vi "EnvCoverRT.vi"(7 "Out limit":bool, 8 "error in (no error)":errorcluster, 9 "ms timeout (0)":i32, 10 "Status in":enum16{"In", "Moving", "Out", "Wait"}(ring), 11 "In limit":bool) -> (0 "error out":errorcluster, 2 "Ready?":bool, 3 "Status out":enum16{"In", "Moving", "Out", "Wait"}(ring))   [LabVIEW 2015]
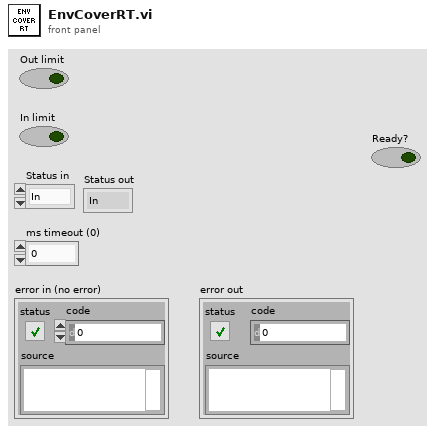
[diagram p1: front panel]
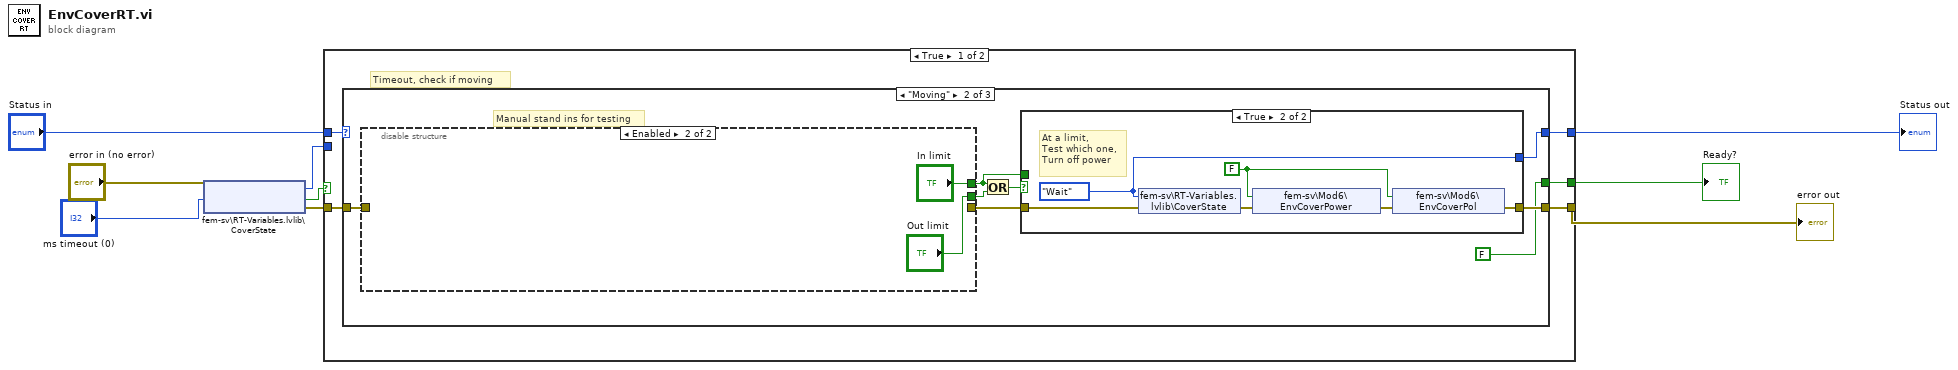
[diagram p0: block diagram]
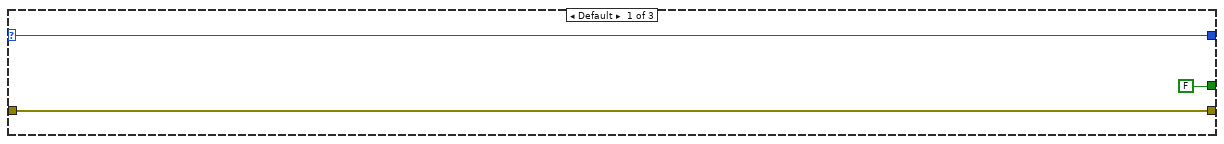
[diagram p2: hidden frame]
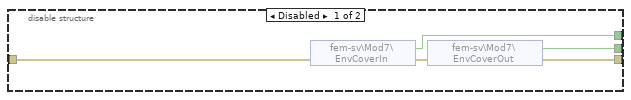
[diagram p3: hidden frame]
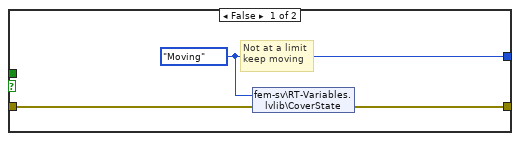
[diagram p4: hidden frame]
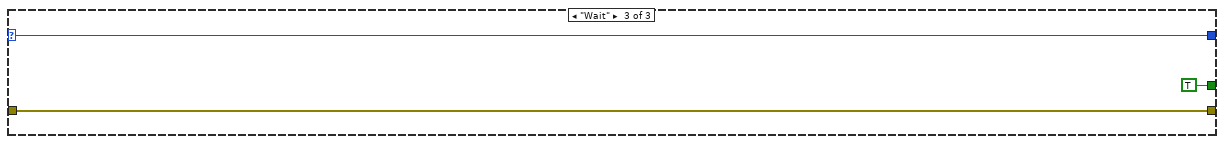
[diagram p5: hidden frame]
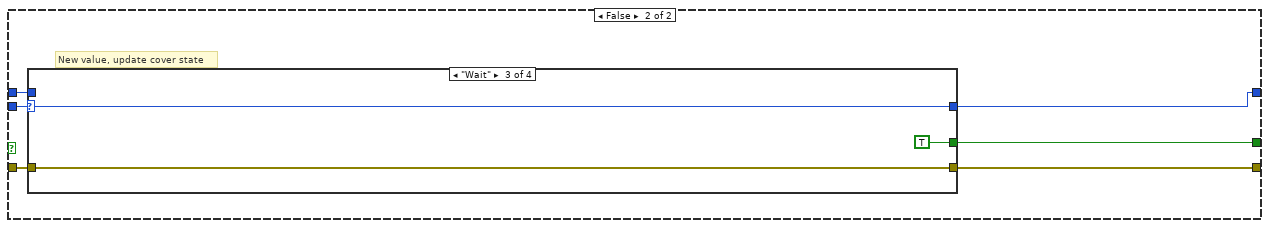
[diagram p6: hidden frame]
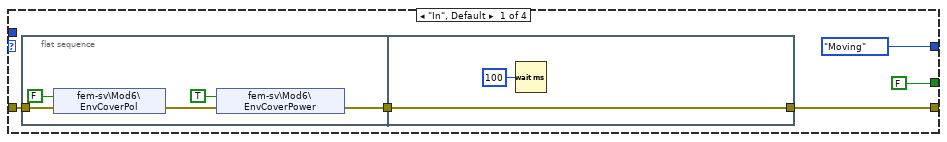
[diagram p7: hidden frame]
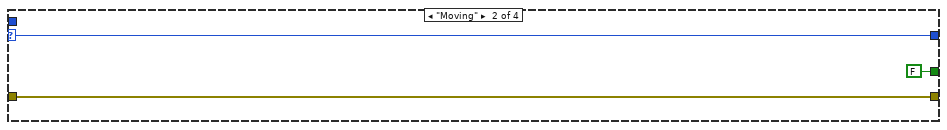
[diagram p8: hidden frame]
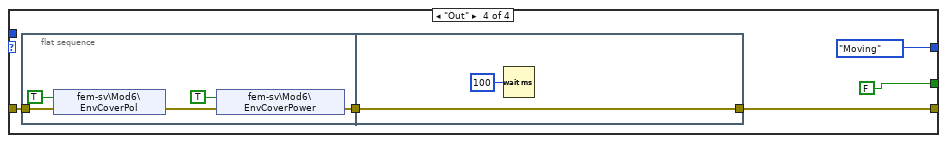
[diagram p9: hidden frame]
diagram:
  n1 = shared-variable "fem-sv\\RT-Variables.lvlib\\CoverState"(error in="error in (no error)", "ms timeout (0)") -> (w5:enum16{"In", "Moving", "Out", "Wait"}, error out=w6:errorcluster, w4:bool)
  n2 = case shown="True" w4 {
    tunnel: [w14 w50] -> w8
    tunnel: "Status in" -> [w11 w49]
    tunnel: w5 -> [_ w48]
    tunnel: w6 -> [w13 w46]
    tunnel: [w12 w47] -> w7
    tunnel: [w10 w45] -> w1
    frame True {
      # "Timeout, check if moving"
      n3 = case shown="\"Moving\"" w11 {
        selector: w11 -> [w17 _ w43]
        tunnel: [w17 w19 w43] -> w14
        tunnel: w13 -> [w16 w23 w42]
        tunnel: [w16 w20 w42] -> w12
        tunnel: [FALSE FALSE TRUE] -> w10
        frame Default {
        }
        frame "Moving" {
          # "Manual stand ins for testing"
          n4 = disable-structure shown="Enabled" {
            disable-tunnel: [w30 "In limit"] -> w24
            disable-tunnel: w23 -> [w29 _]
            disable-tunnel: [w28 "Out limit"] -> w22
            disable-tunnel: [w26 _] -> w21
            frame Disabled {
              n5 = shared-variable "fem-sv\\Mod7\\EnvCoverIn"(error in=w29) -> (w30:bool, error out=w27:errorcluster)
              n6 = shared-variable "fem-sv\\Mod7\\EnvCoverOut"(error in=w27) -> (w28:bool, error out=w26:errorcluster)
            }
            frame Enabled {
            }
          }
          n7 = Or(x=w24, y=w22) -> (x .or. y?=w25:bool)
          n8 = case shown="True" w25 {
            tunnel: w24 -> [_ _]
            tunnel: w21 -> [w35 w41]
            tunnel: [w34 w39] -> w20
            tunnel: [w33 w36] -> w19
            frame False {
              w33 = enum16{"In", "Moving", "Out", "Wait"}."Moving" ("CoverState")
              # "Not at a limit\nkeep moving"
              n9 = shared-variable "fem-sv\\RT-Variables.lvlib\\CoverState"(w33, error in=w35) -> (error out=w34:errorcluster)
            }
            frame True {
              w36 = enum16{"In", "Moving", "Out", "Wait"}."Wait" ("CoverState")
              w37 = FALSE ("EnvCoverPower")
              # "At a limit,\nTest which one,\nTurn off power"
              n10 = shared-variable "fem-sv\\RT-Variables.lvlib\\CoverState"(w36, error in=w41) -> (error out=w38:errorcluster)
              n11 = shared-variable "fem-sv\\Mod6\\EnvCoverPower"(w37, error in=w38) -> (error out=w40:errorcluster)
              n12 = shared-variable "fem-sv\\Mod6\\EnvCoverPol"(w37, error in=w40) -> (error out=w39:errorcluster)
            }
          }
        }
        frame "Wait" {
        }
      }
    }
    frame False {
      # "New value, update cover state"
      n13 = case shown="\"Wait\"" w48 {
        selector: w48 -> [_ w64 w68 _]
        tunnel: [enum16{"In", "Moving", "Out", "Wait"}."Moving" ("Status") w64 w68 enum16{"In", "Moving", "Out", "Wait"}."Moving" ("Status")] -> w50
        tunnel: w49 -> [_ _ _ _]
        tunnel: [w55 w65 w66 w72] -> w47
        tunnel: w46 -> [w54 w65 w66 w73]
        tunnel: [FALSE FALSE TRUE FALSE] -> w45
        frame "In", Default {
          n14 = flat-sequence {
            tunnel: w54 -> [w57]
            tunnel: [w58] -> w52
            tunnel: [w62] -> w55
            tunnel: w52 -> [w62]
            frame #0 {
              n15 = shared-variable "fem-sv\\Mod6\\EnvCoverPol"(FALSE ("EnvCoverPol"), error in=w57) -> (error out=w59:errorcluster)
              n16 = shared-variable "fem-sv\\Mod6\\EnvCoverPower"(TRUE, error in=w59) -> (error out=w58:errorcluster)
            }
            frame #1 {
              n17 = Wait (ms)(milliseconds to wait=u32 100) -> ()  [unwired: 1 out]
            }
          }
        }
        frame "Moving" {
        }
        frame "Wait" {
        }
        frame "Out" {
          n18 = flat-sequence {
            tunnel: w73 -> [w77]
            tunnel: [w76] -> w70
            tunnel: [w80] -> w72
            tunnel: w70 -> [w80]
            frame #0 {
              n19 = shared-variable "fem-sv\\Mod6\\EnvCoverPol"(TRUE ("EnvCoverPol"), error in=w77) -> (error out=w78:errorcluster)
              n20 = shared-variable "fem-sv\\Mod6\\EnvCoverPower"(TRUE ("EnvCoverPower"), error in=w78) -> (error out=w76:errorcluster)
            }
            frame #1 {
              n21 = Wait (ms)(milliseconds to wait=u32 100) -> ()  [unwired: 1 out]
            }
          }
        }
      }
    }
  }
  "Status out" <- w8
  "error out" <- w7
  "Ready?" <- w1
